vi "ReLU_v1.1.2.vi"(1 "x":T1) -> (0 "y":T1)   [LabVIEW 2020]
uses:
  <vilib>/Analysis/Matrix/Datatypes/RealMatrix.ctl
  <vilib>/Analysis/Matrix/Numeric/Conversions/Array To Matrix - RA.vi
  <vilib>/Analysis/Matrix/NI_Matrix.lvlib
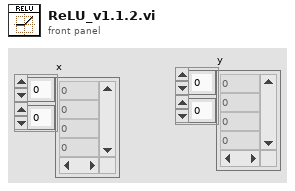
[diagram p1: front panel]
types:
  T1 = typedef "NI_Matrix.lvlib/RealMatrix.ctl" = dbl[][]
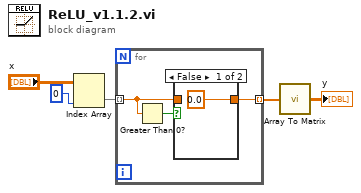
[diagram p0: block diagram]
diagram:
  n1 = Index Array(array="x", index (col)=0) -> (element=w5:dbl[])  [unwired: 1 in]
  n2 = for {
    tunnel: w5 -> [w6] mode=indexing
    tunnel: [w8] -> w4 mode=indexing
    n3 = Greater Than 0?(x=w6) -> (x > 0?=w7:bool)
    n4 = case shown="False" w7 {
      tunnel: w6 -> [_ w10]
      tunnel: [0.0 w10] -> w8
      frame False {
      }
      frame True {
      }
    }
  }
  n5 = call-poly <vilib>:"Array To Matrix.vi"("Real 1D Array"=w4) -> ("Real Matrix (Column Vector)"=→"y":T1)
